vi "Sensorarray_aufloesen.vi"(7 "Array":dbl[](array[numeric])) -> (0 "rechts seite":dbl, 1 "rechts geradeaus":dbl, 2 "rechts Schräg":dbl, 3 "Links schräg":dbl, 4 "Links Geradeaus":dbl, 5 "Links seite":dbl)   [LabVIEW 2016]
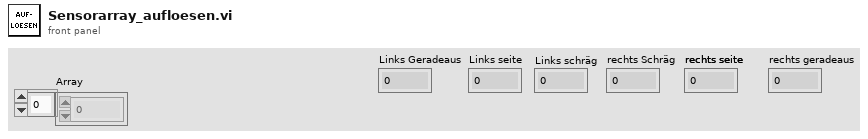
[diagram p1: front panel]
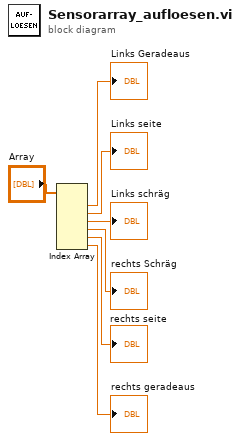
[diagram p0: block diagram]
diagram:
  n1 = Index Array(array="Array") -> (element #1=→"Links Geradeaus":dbl, element #2=→"Links seite":dbl, element #3=→"Links schräg":dbl, element #4=→"rechts Schräg":dbl, element #5=→"rechts seite":dbl, element #6=→"rechts geradeaus":dbl)  [unwired: 6 in]
